vi "Read Openable.vi"(8 "error in (no error)":errorcluster, 11 "Standard VI Type in":refnum<class "Standard VI Type.lvclass">) -> (0 "error out":errorcluster, 2 "Openable?":bool, 3 "Standard VI Type out":refnum<class "Standard VI Type.lvclass">)   [LabVIEW 2020, in "Peek Window.lvlib" / "Standard VI Type.lvclass"]
doc: "Basic read acceessor."
uses:
  Standard VI Type.lvclass
  Standard VI Type.lvclass/Standard VI Type.ctl
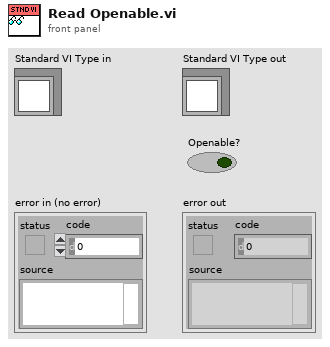
[diagram p1: front panel]
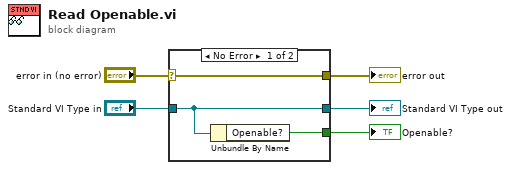
[diagram p0: block diagram]
diagram:
  n1 = case shown="No Error" "error in (no error)" {
    selector: "error in (no error)" -> [w8 w9]
    tunnel: [w8 w9] -> w4
    tunnel: [w7 w10] -> w2
    tunnel: "Standard VI Type in" -> [w7 w10]
    tunnel: [w6 _] -> w1
    frame No Error {
      n2 = Unbundle By Name(w7) -> ("Openable?"=w6:bool)
    }
    frame Error {
    }
  }
  "error out" <- w4
  "Standard VI Type out" <- w2
  "Openable?" <- w1
